vi "GET_url_body.vi"(8 "error in (no error)":errorcluster, 10 "url":string, 11 "comic_class in":refnum<class "comic_class.lvclass">) -> (0 "error out":errorcluster, 2 "body":string, 3 "comic_class out":refnum<class "comic_class.lvclass">)   [LabVIEW 2024, in "comic_class.lvclass"]
uses:
  comic_class.lvclass
  comic_class.lvclass/comic_class.ctl
  <vilib>/httpClient/LabVIEWHTTPClient.lvlib
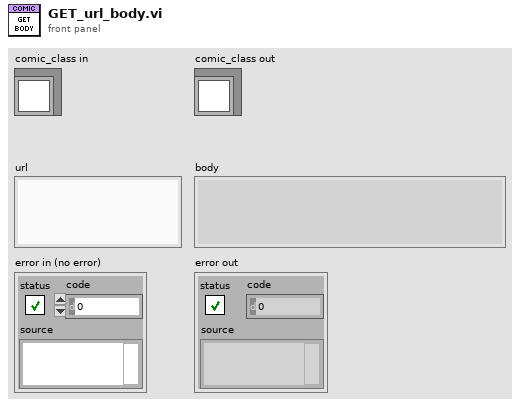
[diagram p1: front panel]
types:
  T1 = typedef "LabVIEWHTTPClient.lvlib/ClientHandle.ctl" = refnum<k1>
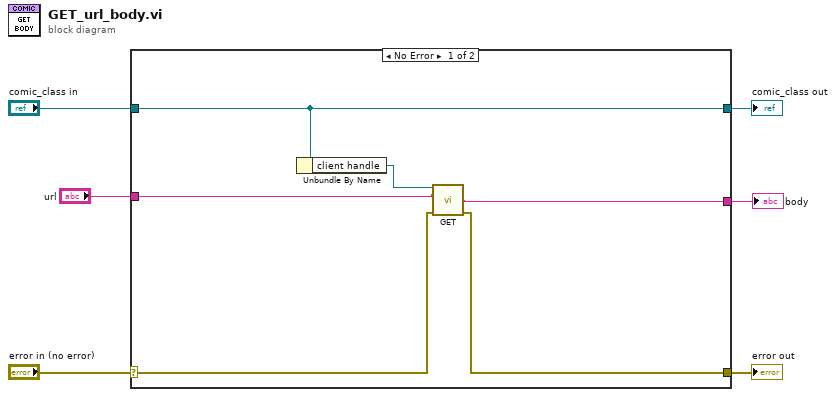
[diagram p0: block diagram]
diagram:
  n1 = case shown="No Error" "error in (no error)" {
    selector: "error in (no error)" -> [w8 w14]
    tunnel: [w7 w14] -> w5
    tunnel: [w11 w13] -> w3
    tunnel: "comic_class in" -> [w11 w13]
    tunnel: "url" -> [w10 _]
    tunnel: [w9 _] -> w1
    frame No Error {
      n2 = Unbundle By Name(w11) -> ("client handle"=w12:T1)
      n3 = call <vilib>:"GET.vi"("client handle"=w12, "url"=w10, "error in (no error)"=w8) -> ("body"=w9:string, "error out"=w7:errorcluster)  [unwired: 9 in, 2 out]
    }
    frame Error {
    }
  }
  "error out" <- w5
  "comic_class out" <- w3
  "body" <- w1
